vi "InActive_Target.vi"(10 "XYGraph Refnum":refnum<vi>) -> (2 "Active Plot":u32)   [LabVIEW 2010]
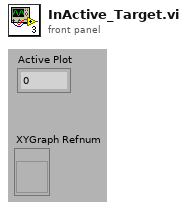
[diagram p1: front panel]
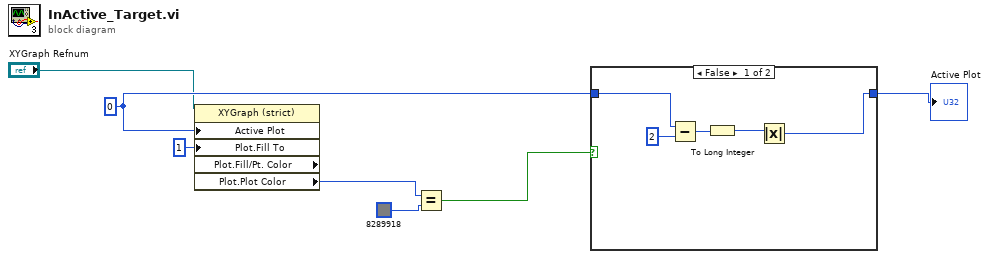
[diagram p0: block diagram]
diagram:
  w6 = u32 0 ("Active Plot")
  n1 = property on="Property Node" class="XYGraph (strict)" props=["Active Plot", "Plot", "Fill To", "Plot", "Fill/Pt. Color", "Plot", "Plot Color"](reference="XYGraph Refnum", "Active Plot"=w6, "Plot.Fill To"=i16 1) -> ("Plot.Plot Color"=w3:u32)  [unwired: 1 in, 3 out]
  n2 = Equal?(x=w3, y=u32 8289918) -> (x = y?=w5:bool)
  n3 = case shown="False" w5 {
    tunnel: w6 -> [w12 w13]
    tunnel: [w8 w13] -> w2
    frame False {
      n4 = Subtract(x=w12, y=u32 2) -> (x-y=w10:u32)
      n5 = To Long Integer(number=w10) -> (32bit integer=w9:i32)
      n6 = Absolute Value(x=w9) -> (abs(x)=w8:i32)
    }
    frame True {
    }
  }
  "Active Plot" <- w2
